vi "BRig_arrTrig_L_ENL2_laser_l1.vi"() -> (2 "output_L_ENL2_laserTrig_l1":i32)   [LabVIEW 2014]
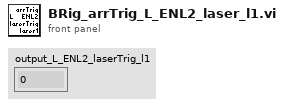
[diagram p1: front panel]
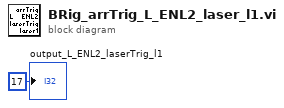
[diagram p0: block diagram]
diagram:
  "output_L_ENL2_laserTrig_l1" <- 17
